vi "ABB Load-Save config.vi"(10 "confirm save":bool, 11 "Mode":enum16{"LOAD", "SAVE"}(ring)) -> ()   [LabVIEW 2017]
uses:
  ABB global.vi
panel:
  out "first row":string[](array[string])
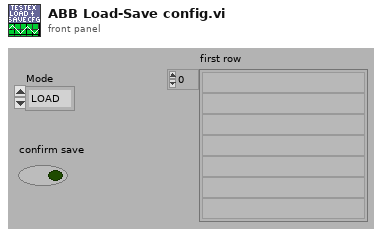
[diagram p1: front panel]
types:
  T1 = cluster{"First row[0]":string, "First row[1]":string, "First row[2]":string, "First row[3]":string}
  T2 = cluster{"First row[0]":string, "First row[1]":string, "First row[2]":string, "First row[3]":string, "First row[4]":string, "First row[5]":string, "First row[6]":string, "First row[7]":string, "First row[8]":string}
  T3 = cluster{"Number Values":i32, "Tolerance":dbl, "Value (ratio) ":dbl[], "Hold time (sec)":dbl}
  T4 = cluster{"Thermal Stability (deg/hr)":dbl, "Reading interval (mins)":dbl}
  T5 = cluster{"Number Values":i32, "Tolerance ":dbl, "Value (ratio)":dbl[], "Hold time (sec)":dbl}
  T6 = cluster{"Simulate Norma":bool, "Norma 5000 Address":u8, "WebDaq IP Address":string, "Simulate cDAQ":bool}
  T7 = cluster{"temp. alloc":i32[], "category":i32[], "Category names":string[], "Category none names":string[]}
  T8 = cluster{"Number of Loads":i32, "Loads (%Rated)":dbl[]}
  T9 = cluster{"VT Primary":dbl, "VT Secondary":dbl, "CT  Primary":dbl, "CT Secondary":dbl, "Current Shunt":enum16{"Internal", "External"}, "Averaging interval":dbl}
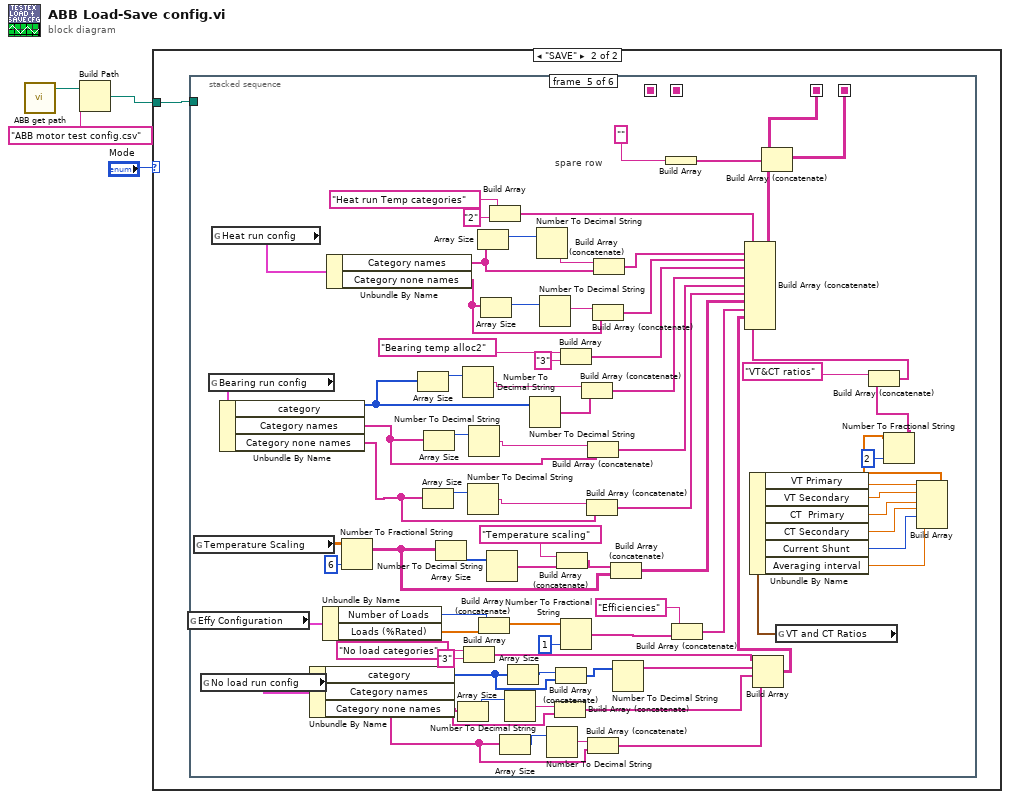
[diagram p0: block diagram]
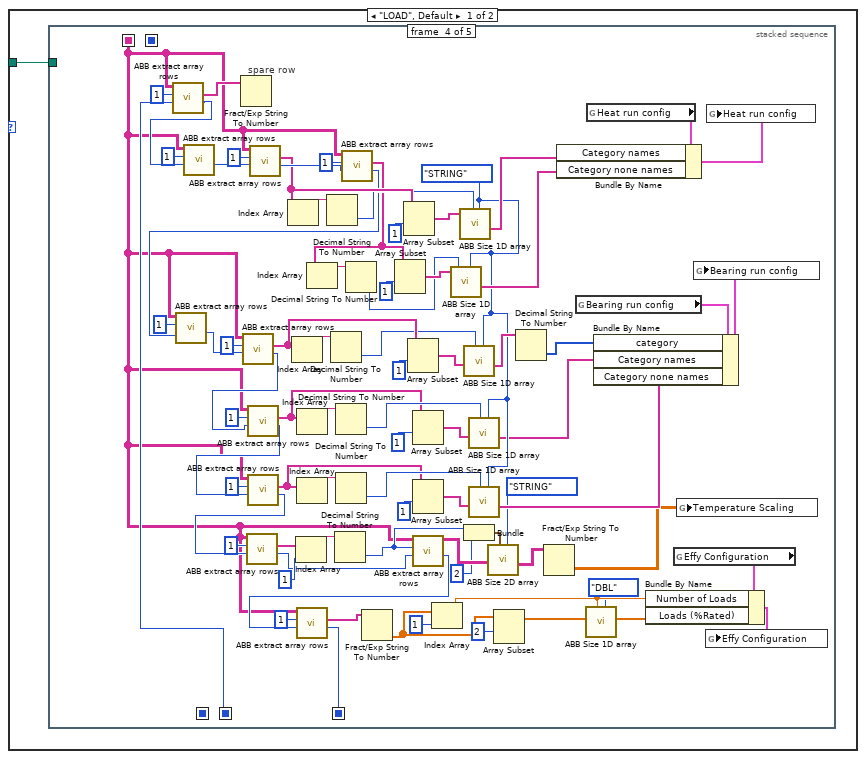
[diagram p2: hidden frame]
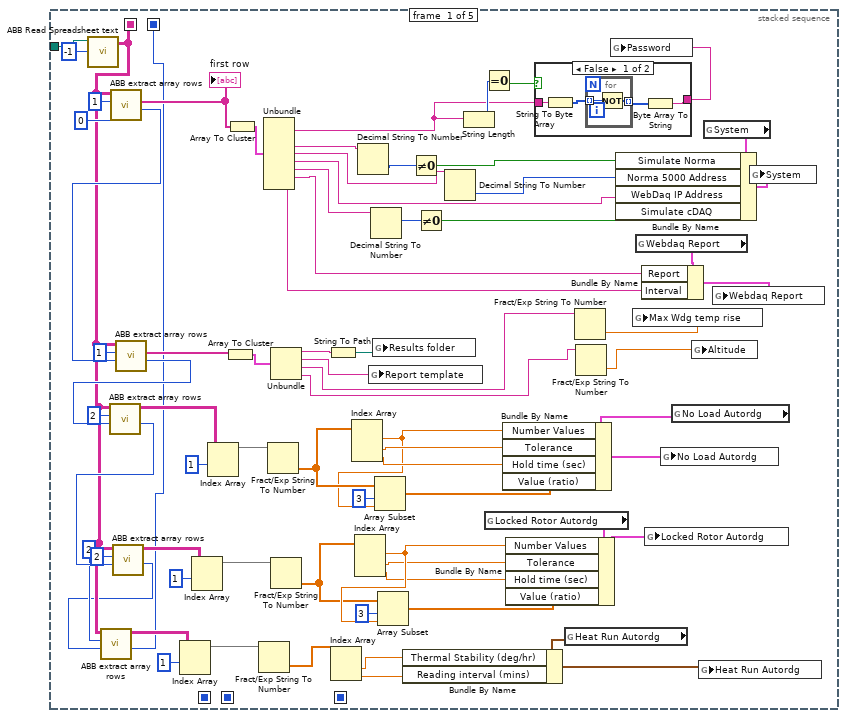
[diagram p3: hidden frame]
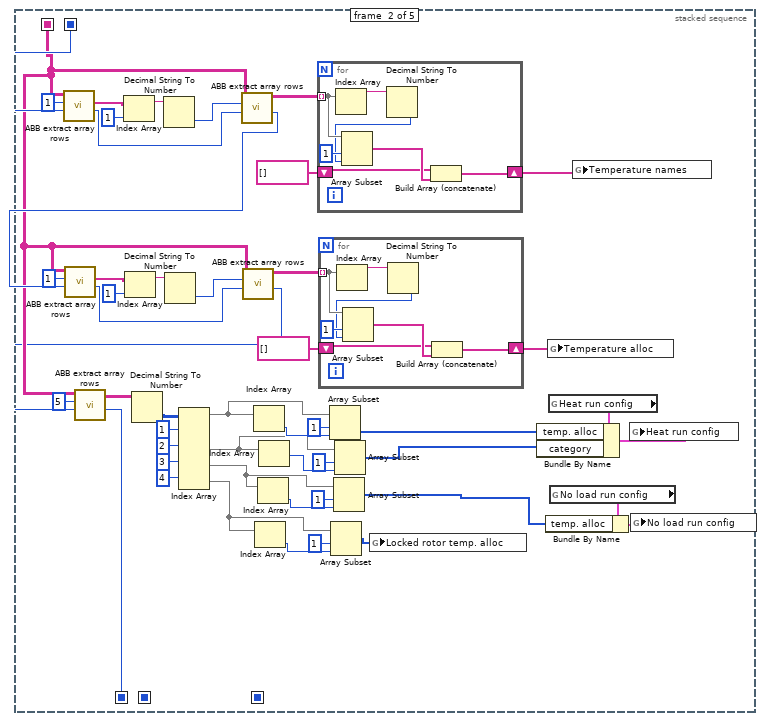
[diagram p5: hidden frame]
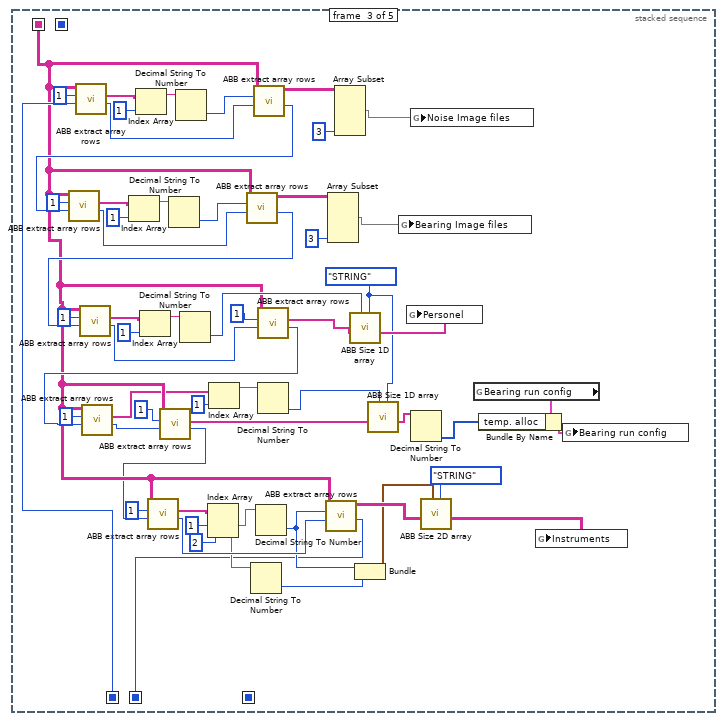
[diagram p6: hidden frame]
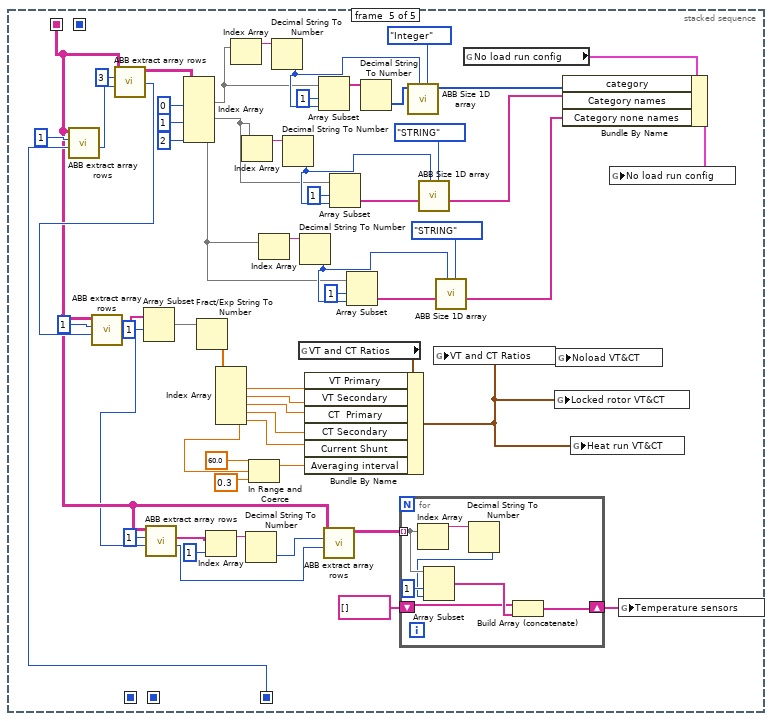
[diagram p7: hidden frame]
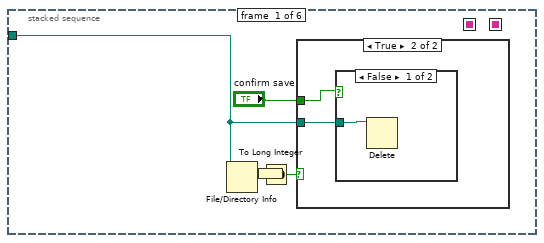
[diagram p8: hidden frame]
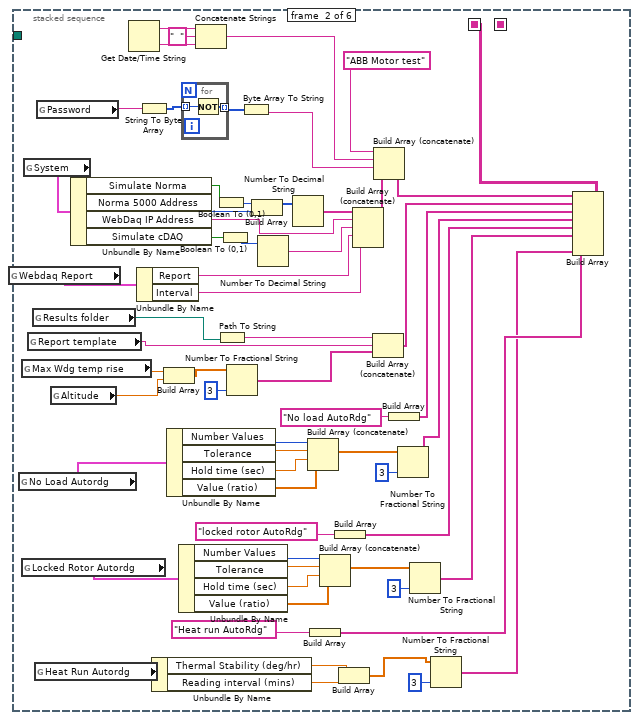
[diagram p11: hidden frame]
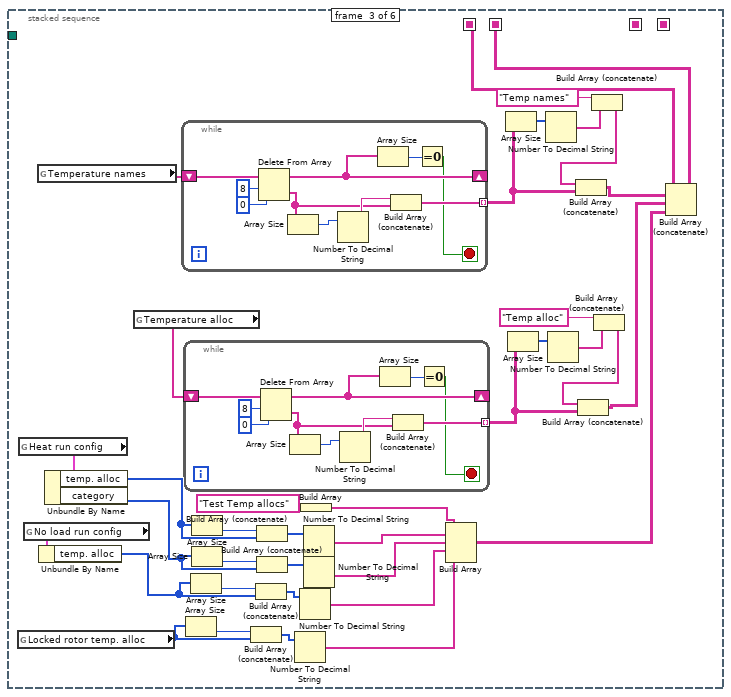
[diagram p12: hidden frame]
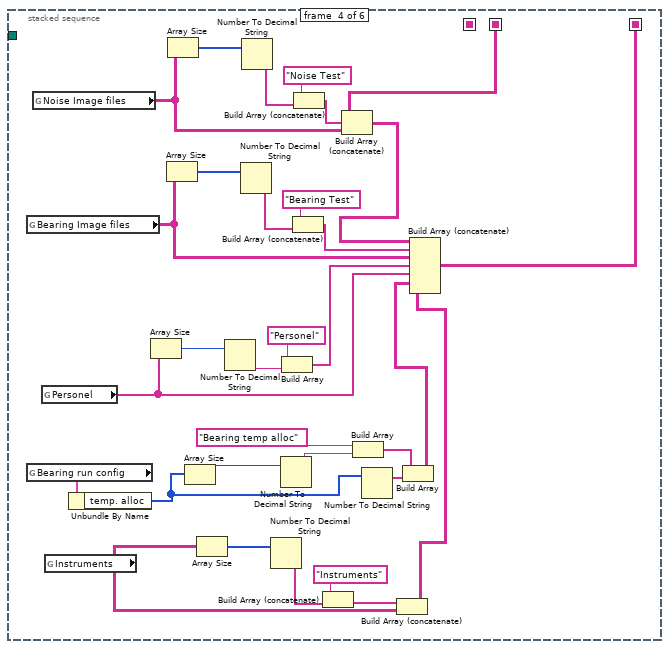
[diagram p13: hidden frame]
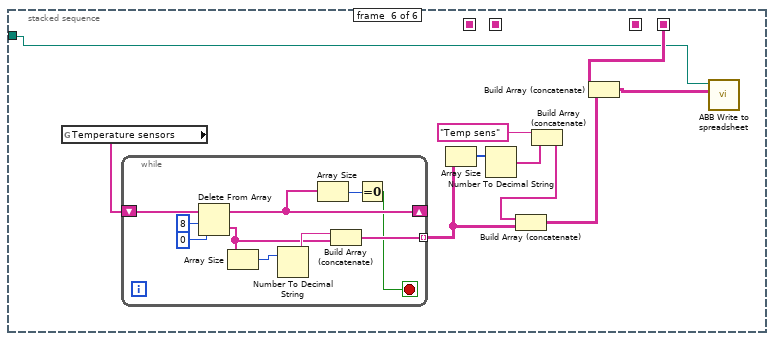
[diagram p14: hidden frame]
diagram:
  n1 = call "ABB get path.vi"() -> ("Path"=w1:path)  [unwired: 11 in]
  n2 = Build Path(base path=w1, name or relative path="ABB motor test config.csv") -> (appended path=w2:path)
  n3 = case shown="\"SAVE\"" "Mode" {
    tunnel: w2 -> [w5 w357]
    frame "LOAD", Default {
      n4 = stacked-sequence {
        seq-local: [w27 _ _ _ _] -> [_ w115 w159 w212 w292]
        seq-local: [w20 _ _ _ _] -> [_ w135 _ _ _]
        seq-local: [_ w100 _ _ _] -> [_ _ w204 _ _]
        seq-local: [_ _ w163 _ _] -> [_ _ _ w289 _]
        seq-local: [_ _ _ w211 _] -> [_ _ _ _ w348]
        tunnel: w5 -> [w74 _ _ _ _]
        frame #0 {
          n5 = call "ABB Read Spreadsheet text.vi"("number of rows (all:-1)"=-1, "file path (dialog if empty)"=w74) -> ("all rows"=w27:string[][])  [unwired: 5 in, 4 out]
          n6 = call "ABB extract array rows.vi"("Row offset"=0, "# rows"=1, "Input array"=w27) -> ("Next row"=w62:i32, "First row"=w71:string[])  [unwired: 6 in, 1 out]
          "first row" <- w71
          n7 = call "ABB extract array rows.vi"("Row offset"=w62, "# rows"=1, "Input array"=w27) -> ("Next row"=w56:i32, "First row"=w61:string[])  [unwired: 6 in, 1 out]
          n8 = call "ABB extract array rows.vi"("Row offset"=w56, "# rows"=2, "Input array"=w27) -> ("Next row"=w32:i32, "All rows"=w55:string[][])  [unwired: 6 in, 1 out]
          n9 = call "ABB extract array rows.vi"("Row offset"=w32, "# rows"=2, "Input array"=w27) -> ("Next row"=w26:i32, "All rows"=w34:string[][])  [unwired: 6 in, 1 out]
          n10 = call "ABB extract array rows.vi"("Row offset"=w26, "# rows"=2, "Input array"=w27) -> ("Next row"=w20:i32, "All rows"=w30:string[][])  [unwired: 6 in, 1 out]
          n11 = Index Array(array=w30, index (row)=1) -> (element=w28:string[])  [unwired: 1 in]
          n12 = Index Array(array=w34, index (row)=1) -> (element=w36:string[])  [unwired: 1 in]
          n13 = Index Array(array=w55, index (row)=1) -> (element=w53:string[])  [unwired: 1 in]
          n14 = Array To Cluster(array=w61) -> (cluster=w60:T1)
          n15 = Array To Cluster(array=w71) -> (cluster=w79:T2)
          n16 = Fract/Exp String To Number(string=w28) -> (number=w24:dbl[])  [unwired: 3 in, 1 out]
          n17 = Unbundle(w79) -> ("First row[2]"=w73:string, "First row[3]"=w69:string, "First row[4]"=w18:string, "First row[5]"=w17:string, "First row[6]"=w16:string, "First row[7]"=w6:string, "First row[8]"=w7:string)  [unwired: 2 out]
          n18 = Fract/Exp String To Number(string=w53) -> (number=w49:dbl[])  [unwired: 3 in, 1 out]
          n19 = Unbundle(w60) -> ("First row[0]"=w59:string, "First row[1]"=w19:string, "First row[2]"=w13:string, "First row[3]"=w12:string)
          n20 = Fract/Exp String To Number(string=w36) -> (number=w40:dbl[])  [unwired: 3 in, 1 out]
          n21 = String To Path(string=w59) -> (path=w58:path)
          n22 = Index Array(array=w24) -> (element #1=w23:dbl, element #2=w22:dbl)  [unwired: 2 in]
          n23 = Index Array(array=w49) -> (element #1=w47:dbl, element #2=w51:dbl, element #3=w50:dbl)  [unwired: 3 in]
          n24 = Index Array(array=w40) -> (element #1=w42:dbl, element #2=w38:dbl, element #3=w39:dbl)  [unwired: 3 in]
          n25 = Decimal String To Number(string=w69) -> (number=w68:i32)  [unwired: 2 in, 1 out]
          n26 = global write "ABB global.vi" "Report template"(w19) -> ()
          n27 = Decimal String To Number(string=w16) -> (number=w15:i32)  [unwired: 2 in, 1 out]
          n28 = global write "ABB global.vi" "Results folder"(w58) -> ()
          n29 = Array Subset(array=w49, index=3, length=w47) -> (w46:dbl[])
          n30 = Array Subset(array=w40, index=3, length=w42) -> (w43:dbl[])
          n31 = Not Equal To 0?(x=w68) -> (x != 0?=w66:bool)
          n32 = Not Equal To 0?(x=w15) -> (x != 0?=w14:bool)
          n33 = Decimal String To Number(string=w18) -> (number=w65:i32)  [unwired: 2 in, 1 out]
          n34 = String Length(string=w73) -> (length=w78:i32)
          n35 = Equal To 0?(x=w78) -> (x = 0?=w77:bool)
          n36 = global read "ABB global.vi" "Locked Rotor Autordg"() -> (w37:T3)
          n37 = Bundle By Name(cluster=w37, "Number Values"=w42, "Tolerance"=w38, "Hold time (sec)"=w39, "Value (ratio)"=w43) -> (w44:T3)
          n38 = case shown="False" w77 {
            tunnel: w73 -> [w81 w86]
            tunnel: [w80 w86] -> w76
            frame False {
              n39 = String To Byte Array(string=w81) -> (unsigned byte array=w83:u8[])
              n40 = for {
                tunnel: w83 -> [w85] mode=indexing
                tunnel: [w84] -> w82 mode=indexing
                n41 = Not(x=w85) -> (.not. x?=w84:u8)
              }
              n42 = Byte Array To String(unsigned byte array=w82) -> (string=w80:string)
            }
            frame True {
            }
          }
          n43 = global read "ABB global.vi" "Heat Run Autordg"() -> (w25:T4)
          n44 = Bundle By Name(cluster=w25, "Thermal Stability (deg/hr)"=w23, "Reading interval (mins)"=w22) -> (w21:T4)
          n45 = Fract/Exp String To Number(string=w13) -> (number=w11:dbl)  [unwired: 3 in, 1 out]
          n46 = Fract/Exp String To Number(string=w12) -> (number=w10:dbl)  [unwired: 3 in, 1 out]
          n47 = global write "ABB global.vi" "Password"(w76) -> ()
          n48 = global write "ABB global.vi" "Max Wdg temp rise"(w11) -> ()
          n49 = global read "ABB global.vi" "Webdaq Report"() -> (w9:cluster{"Report":string, "Interval":string})
          n50 = Bundle By Name(cluster=w9, "Report"=w6, "Interval"=w7) -> (w8:cluster{"Report":string, "Interval":string})
          n51 = global write "ABB global.vi" "Locked Rotor Autordg"(w44) -> ()
          n52 = global read "ABB global.vi" "No Load Autordg"() -> (w52:T5)
          n53 = Bundle By Name(cluster=w52, "Number Values"=w47, "Tolerance"=w51, "Hold time (sec)"=w50, "Value (ratio)"=w46) -> (w45:T5)
          n54 = global write "ABB global.vi" "No Load Autordg"(w45) -> ()
          n55 = global write "ABB global.vi" "Altitude"(w10) -> ()
          n56 = global write "ABB global.vi" "Heat Run Autordg"(w21) -> ()
          n57 = global read "ABB global.vi" "System"() -> (w67:T6)
          n58 = Bundle By Name(cluster=w67, "Simulate Norma"=w66, "Norma 5000 Address"=w65, "WebDaq IP Address"=w17, "Simulate cDAQ"=w14) -> (w64:T6)
          n59 = global write "ABB global.vi" "Webdaq Report"(w8) -> ()
          n60 = global write "ABB global.vi" "System"(w64) -> ()
        }
        frame #1 {
          n61 = call "ABB extract array rows.vi"("Row offset"=w135, "# rows"=1, "Input array"=w115) -> ("Next row"=w131:i32, "First row"=w134:string[])  [unwired: 6 in, 1 out]
          n62 = Index Array(array=w134, index=1) -> (element=w132:string)
          n63 = Decimal String To Number(string=w132) -> (number=w130:i32)  [unwired: 2 in, 1 out]
          n64 = call "ABB extract array rows.vi"("Row offset"=w131, "# rows"=w130, "Input array"=w115) -> ("Next row"=w118:i32, "All rows"=w129:string[][])  [unwired: 6 in, 1 out]
          n65 = call "ABB extract array rows.vi"("Row offset"=w118, "# rows"=1, "Input array"=w115) -> ("Next row"=w123:i32, "First row"=w120:string[])  [unwired: 6 in, 1 out]
          n66 = Index Array(array=w120, index=1) -> (element=w122:string)
          n67 = Decimal String To Number(string=w122) -> (number=w124:i32)  [unwired: 2 in, 1 out]
          n68 = call "ABB extract array rows.vi"("Row offset"=w123, "# rows"=w124, "Input array"=w115) -> ("Next row"=w109:i32, "All rows"=w125:string[][])  [unwired: 6 in, 1 out]
          n69 = call "ABB extract array rows.vi"("Row offset"=w109, "# rows"=5, "Input array"=w115) -> ("Next row"=w100:i32, "All rows"=w114:string[][])  [unwired: 6 in, 1 out]
          n70 = Decimal String To Number(string=w114) -> (number=w113:i32[][])  [unwired: 2 in, 1 out]
          n71 = Index Array(array=w113, index (row) #1=1 ("index (row)"), index (row) #2=2 ("index (row)"), index (row) #3=3 ("index (row)"), index (row) #4=4 ("index (row)")) -> (element #1=w107:i32[], element #2=w94:i32[], element #3=w92:i32[], element #4=w91:i32[])  [unwired: 4 in]
          n72 = Index Array(array=w107) -> (element=w108:i32)  [unwired: 1 in]
          n73 = Index Array(array=w91) -> (element=w103:i32)  [unwired: 1 in]
          n74 = Index Array(array=w92) -> (element=w104:i32)  [unwired: 1 in]
          n75 = Index Array(array=w94) -> (element=w90:i32)  [unwired: 1 in]
          n76 = for {
            tunnel: w129 -> [w150] mode=indexing
            shift-right: [w144] -> w127
            shift-left: string[] [] -> [w145]
            n77 = Index Array(array=w150) -> (element=w148:string)  [unwired: 1 in]
            n78 = Decimal String To Number(string=w148) -> (number=w147:i32)  [unwired: 2 in, 1 out]
            n79 = Array Subset(array=w150, index=1, length=w147) -> (w146:string[])
            n80 = Build Array (concatenate)(w145, w146) -> (w144:string[])
          }
          n81 = for {
            tunnel: w125 -> [w143] mode=indexing
            shift-right: [w137] -> w117
            shift-left: string[] [] -> [w138]
            n82 = Index Array(array=w143) -> (element=w141:string)  [unwired: 1 in]
            n83 = Decimal String To Number(string=w141) -> (number=w140:i32)  [unwired: 2 in, 1 out]
            n84 = Array Subset(array=w143, index=1, length=w140) -> (w139:string[])
            n85 = Build Array (concatenate)(w138, w139) -> (w137:string[])
          }
          n86 = Array Subset(array=w107, index=1, length=w108) -> (w97:i32[])
          n87 = Array Subset(array=w91, index=1, length=w103) -> (w101:i32[])
          n88 = Array Subset(array=w92, index=1, length=w104) -> (w87:i32[])
          n89 = Array Subset(array=w94, index=1, length=w90) -> (w93:i32[])
          n90 = global write "ABB global.vi" "Locked rotor temp. alloc"(w101) -> ()
          n91 = global write "ABB global.vi" "Temperature alloc"(w117) -> ()
          n92 = global read "ABB global.vi" "Heat run config"() -> (w99:T7)
          n93 = Bundle By Name(cluster=w99, "temp. alloc"=w97, "category"=w93) -> (w98:T7)
          n94 = global read "ABB global.vi" "No load run config"() -> (w88:T7)
          n95 = Bundle By Name(cluster=w88, "temp. alloc"=w87) -> (w89:T7)
          n96 = global write "ABB global.vi" "Temperature names"(w127) -> ()
          n97 = global write "ABB global.vi" "Heat run config"(w98) -> ()
          n98 = global write "ABB global.vi" "No load run config"(w89) -> ()
        }
        frame #2 {
          w178 = enum16{"Integer", "DBL", "STRING", "BOOLEAN"}."STRING" ("Type")
          n99 = call "ABB extract array rows.vi"("Row offset"=w204, "# rows"=1, "Input array"=w159) -> ("Next row"=w209:i32, "First row"=w206:string[])  [unwired: 6 in, 1 out]
          n100 = Index Array(array=w206, index=1) -> (element=w208:string)
          n101 = Decimal String To Number(string=w208) -> (number=w210:i32)  [unwired: 2 in, 1 out]
          n102 = call "ABB extract array rows.vi"("Row offset"=w209, "# rows"=w210, "Input array"=w159) -> ("Next row"=w191:i32, "All rows"=w203:string[][])  [unwired: 6 in, 1 out]
          n103 = call "ABB extract array rows.vi"("Row offset"=w191, "# rows"=1, "Input array"=w159) -> ("Next row"=w193:i32, "First row"=w196:string[])  [unwired: 6 in, 1 out]
          n104 = Index Array(array=w196, index=1) -> (element=w194:string)
          n105 = Decimal String To Number(string=w194) -> (number=w192:i32)  [unwired: 2 in, 1 out]
          n106 = call "ABB extract array rows.vi"("Row offset"=w193, "# rows"=w192, "Input array"=w159) -> ("Next row"=w186:i32, "All rows"=w198:string[][])  [unwired: 6 in, 1 out]
          n107 = call "ABB extract array rows.vi"("Row offset"=w186, "# rows"=1, "Input array"=w159) -> ("Next row"=w182:i32, "First row"=w188:string[])  [unwired: 6 in, 1 out]
          n108 = Index Array(array=w188, index=1) -> (element=w190:string)
          n109 = Decimal String To Number(string=w190) -> (number=w179:i32)  [unwired: 2 in, 1 out]
          n110 = call "ABB extract array rows.vi"("Row offset"=w182, "# rows"=1, "Input array"=w159) -> ("Next row"=w184:i32, "First row"=w181:string[])  [unwired: 6 in, 1 out]
          n111 = call "ABB extract array rows.vi"("Row offset"=w184, "# rows"=1, "Input array"=w159) -> ("Next row"=w158:i32, "First row"=w154:string[])  [unwired: 6 in, 1 out]
          n112 = call "ABB extract array rows.vi"("Row offset"=w158, "# rows"=1, "Input array"=w159) -> ("Next row"=w157:i32, "First row"=w155:string[])  [unwired: 6 in, 1 out]
          n113 = call "ABB extract array rows.vi"("Row offset"=w157, "# rows"=1, "Input array"=w159) -> ("Next row"=w176:i32, "First row"=w173:string[])  [unwired: 6 in, 1 out]
          n114 = Index Array(array=w173, index #1=1 ("index"), index #2=2 ("index")) -> (element #1=w175:string, element #2=w168:string)
          n115 = Index Array(array=w154, index=1) -> (element=w152:string)
          n116 = Decimal String To Number(string=w168) -> (number=w166:i32)  [unwired: 2 in, 1 out]
          n117 = Decimal String To Number(string=w175) -> (number=w167:i32)  [unwired: 2 in, 1 out]
          n118 = Decimal String To Number(string=w152) -> (number=w151:i32)  [unwired: 2 in, 1 out]
          n119 = call "ABB extract array rows.vi"("Row offset"=w176, "# rows"=w167, "Input array"=w159) -> ("Next row"=w163:i32, "All rows"=w171:string[][])  [unwired: 6 in, 1 out]
          n120 = Array Subset(array=w198, length (col)=3 ("length")) -> (w200:string[][])  [unwired: 3 in]
          n121 = Array Subset(array=w203, length (col)=3 ("length")) -> (w201:string[][])  [unwired: 3 in]
          n122 = call "ABB Size 1D array.vi"("Type"=w178, "Size"=w179, "String Array in"=w181) -> ("String Array out"=w180:string[])  [unwired: 5 in, 3 out]
          n123 = Bundle(w167, w166) -> (w165:cluster{i32, i32})  [unwired: 1 in]
          n124 = call "ABB Size 1D array.vi"("Type"=w178, "Size"=w151, "String Array in"=w155) -> ("String Array out"=w177:string[])  [unwired: 5 in, 3 out]
          n125 = global write "ABB global.vi" "Bearing Image files"(w200) -> ()
          n126 = global write "ABB global.vi" "Personel"(w180) -> ()
          n127 = global write "ABB global.vi" "Noise Image files"(w201) -> ()
          n128 = Decimal String To Number(string=w177) -> (number=w161:i32[])  [unwired: 2 in, 1 out]
          n129 = call "ABB Size 2D array.vi"("Type"=enum16{"Integer", "DBL", "STRING", "BOOLEAN"}."STRING", "Size"=w165, "String Array in"=w171) -> ("String Array out"=w164:string[][])  [unwired: 5 in, 3 out]
          n130 = global read "ABB global.vi" "Bearing run config"() -> (w162:T7)
          n131 = Bundle By Name(cluster=w162, "temp. alloc"=w161) -> (w160:T7)
          n132 = global write "ABB global.vi" "Instruments"(w164) -> ()
          n133 = global write "ABB global.vi" "Bearing run config"(w160) -> ()
        }
        frame #3 {
          w240 = enum16{"Integer", "DBL", "STRING", "BOOLEAN"}."STRING" ("Type")
          # "spare row"
          n134 = call "ABB extract array rows.vi"("Row offset"=w289, "# rows"=1, "Input array"=w212) -> ("Next row"=w282:i32, "First row"=w288:string[])  [unwired: 6 in, 1 out]
          n135 = call "ABB extract array rows.vi"("Row offset"=w282, "# rows"=1, "Input array"=w212) -> ("Next row"=w281:i32)  [unwired: 6 in, 2 out]
          n136 = Fract/Exp String To Number(string=w288) -> ()  [unwired: 3 in, 2 out]
          n137 = call "ABB extract array rows.vi"("Row offset"=w281, "# rows"=1, "Input array"=w212) -> ("Next row"=w280:i32, "First row"=w278:string[])  [unwired: 6 in, 1 out]
          n138 = Index Array(array=w278) -> (element=w279:string)  [unwired: 1 in]
          n139 = Decimal String To Number(string=w279) -> (number=w274:i32)  [unwired: 2 in, 1 out]
          n140 = call "ABB extract array rows.vi"("Row offset"=w280, "# rows"=1, "Input array"=w212) -> ("Next row"=w262:i32, "First row"=w270:string[])  [unwired: 6 in, 1 out]
          n141 = call "ABB extract array rows.vi"("Row offset"=w262, "# rows"=1, "Input array"=w212) -> ("Next row"=w265:i32)  [unwired: 6 in, 2 out]
          n142 = call "ABB extract array rows.vi"("Row offset"=w265, "# rows"=1, "Input array"=w212) -> ("Next row"=w244:i32, "First row"=w259:string[])  [unwired: 6 in, 1 out]
          n143 = call "ABB extract array rows.vi"("Row offset"=w244, "# rows"=1, "Input array"=w212) -> ("Next row"=w243:i32, "First row"=w242:string[])  [unwired: 6 in, 1 out]
          n144 = call "ABB extract array rows.vi"("Row offset"=w243, "# rows"=1, "Input array"=w212) -> ("Next row"=w234:i32, "First row"=w241:string[])  [unwired: 6 in, 1 out]
          n145 = call "ABB extract array rows.vi"("Row offset"=w234, "# rows"=1, "Input array"=w212) -> ("Next row"=w232:i32, "First row"=w237:string[])  [unwired: 6 in, 1 out]
          n146 = Index Array(array=w259) -> (element=w257:string)  [unwired: 1 in]
          n147 = Index Array(array=w237, index=1) -> (element=w236:string)
          n148 = Index Array(array=w242) -> (element=w254:string)  [unwired: 1 in]
          n149 = Index Array(array=w241) -> (element=w245:string)  [unwired: 1 in]
          n150 = Index Array(array=w270) -> (element=w271:string)  [unwired: 1 in]
          n151 = Decimal String To Number(string=w257) -> (number=w258:i32)  [unwired: 2 in, 1 out]
          n152 = Decimal String To Number(string=w236) -> (number=w229:i32)  [unwired: 2 in, 1 out]
          n153 = Decimal String To Number(string=w254) -> (number=w253:i32)  [unwired: 2 in, 1 out]
          n154 = Decimal String To Number(string=w245) -> (number=w246:i32)  [unwired: 2 in, 1 out]
          n155 = Decimal String To Number(string=w271) -> (number=w269:i32)  [unwired: 2 in, 1 out]
          n156 = Array Subset(array=w270, index=1) -> (w273:string[])  [unwired: 1 in]
          n157 = Array Subset(array=w278, index=1) -> (w276:string[])  [unwired: 1 in]
          n158 = Array Subset(array=w259, index=1) -> (w261:string[])  [unwired: 1 in]
          n159 = Array Subset(array=w242, index=1) -> (w251:string[])  [unwired: 1 in]
          n160 = Array Subset(array=w241, index=1) -> (w248:string[])  [unwired: 1 in]
          n161 = call "ABB extract array rows.vi"("Row offset"=w232, "# rows"=w229, "Input array"=w212) -> ("Next row"=w223:i32, "All rows"=w231:string[][])  [unwired: 6 in, 1 out]
          n162 = call "ABB extract array rows.vi"("Row offset"=w223, "# rows"=1, "Input array"=w212) -> ("Next row"=w211:i32, "First row"=w222:string[])  [unwired: 6 in, 1 out]
          n163 = Fract/Exp String To Number(string=w222) -> (number=w220:dbl[])  [unwired: 3 in, 1 out]
          n164 = Index Array(array=w220, index=1) -> (element=w216:dbl)
          n165 = call "ABB Size 1D array.vi"("Type"=w240, "Size"=w269, "String Array in"=w273) -> ("String Array out"=w268:string[])  [unwired: 5 in, 3 out]
          n166 = call "ABB Size 1D array.vi"("Type"=w240, "Size"=w274, "String Array in"=w276) -> ("String Array out"=w275:string[])  [unwired: 5 in, 3 out]
          n167 = call "ABB Size 1D array.vi"("Type"=w240, "Size"=w258, "String Array in"=w261) -> ("String Array out"=w256:string[])  [unwired: 5 in, 3 out]
          n168 = Bundle(w229, 2) -> (w227:cluster{i32, i32})  [unwired: 1 in]
          n169 = call "ABB Size 1D array.vi"("Type"=w240, "Size"=w253, "String Array in"=w251) -> ("String Array out"=w238:string[])  [unwired: 5 in, 3 out]
          n170 = call "ABB Size 1D array.vi"("Type"=w240, "Size"=w246, "String Array in"=w248) -> ("String Array out"=w239:string[])  [unwired: 5 in, 3 out]
          n171 = call "ABB Size 2D array.vi"("Type"=enum16{"Integer", "DBL", "STRING", "BOOLEAN"}."STRING", "Size"=w227, "String Array in"=w231) -> ("String Array out"=w226:string[][])  [unwired: 5 in, 3 out]
          n172 = Array Subset(array=w220, index=2) -> (w217:dbl[])  [unwired: 1 in]
          n173 = Decimal String To Number(string=w256) -> (number=w255:i32[])  [unwired: 2 in, 1 out]
          n174 = Fract/Exp String To Number(string=w226) -> (number=w225:dbl[][])  [unwired: 3 in, 1 out]
          n175 = global read "ABB global.vi" "Bearing run config"() -> (w267:T7)
          n176 = call "ABB Size 1D array.vi"("Type"=enum16{"Integer", "DBL", "STRING", "BOOLEAN"}."DBL", "Size"=w216, "DBL Array In"=w217) -> ("DBL Array out"=w213:dbl[])  [unwired: 5 in, 3 out]
          n177 = global read "ABB global.vi" "Heat run config"() -> (w287:T7)
          n178 = Bundle By Name(cluster=w287, "Category names"=w275, "Category none names"=w268) -> (w286:T7)
          n179 = Bundle By Name(cluster=w267, "category"=w255, "Category names"=w238, "Category none names"=w239) -> (w266:T7)
          n180 = global read "ABB global.vi" "Effy Configuration"() -> (w218:T8)
          n181 = Bundle By Name(cluster=w218, "Number of Loads"=w216, "Loads (%Rated)"=w213) -> (w214:T8)
          n182 = global write "ABB global.vi" "Temperature Scaling"(w225) -> ()
          n183 = global write "ABB global.vi" "Bearing run config"(w266) -> ()
          n184 = global write "ABB global.vi" "Effy Configuration"(w214) -> ()
          n185 = global write "ABB global.vi" "Heat run config"(w286) -> ()
        }
        frame #4 {
          n186 = call "ABB extract array rows.vi"("Row offset"=w348, "# rows"=1, "Input array"=w292) -> ("Next row"=w346:i32)  [unwired: 6 in, 2 out]
          n187 = call "ABB extract array rows.vi"("Row offset"=w346, "# rows"=3, "Input array"=w292) -> ("Next row"=w316:i32, "All rows"=w336:string[][])  [unwired: 6 in, 1 out]
          n188 = call "ABB extract array rows.vi"("Row offset"=w316, "# rows"=1, "Input array"=w292) -> ("Next row"=w291:i32, "First row"=w308:string[])  [unwired: 6 in, 1 out]
          n189 = Array Subset(array=w308, index=1) -> (w309:string[])  [unwired: 1 in]
          n190 = call "ABB extract array rows.vi"("Row offset"=w291, "# rows"=1, "Input array"=w292) -> ("Next row"=w298:i32, "First row"=w295:string[])  [unwired: 6 in, 1 out]
          n191 = Index Array(array=w336, index (row) #1=0 ("index (row)"), index (row) #2=1 ("index (row)"), index (row) #3=2 ("index (row)")) -> (element #1=w335:string[], element #2=w323:string[], element #3=w318:string[])  [unwired: 3 in]
          n192 = Fract/Exp String To Number(string=w309) -> (number=w314:dbl[])  [unwired: 3 in, 1 out]
          n193 = Index Array(array=w295, index=1) -> (element=w297:string)
          n194 = Index Array(array=w314) -> (element #1=w313:dbl, element #2=w312:dbl, element #3=w311:dbl, element #4=w310:dbl, element #5=w305:dbl)  [unwired: 5 in]
          n195 = Index Array(array=w335) -> (element=w345:string)  [unwired: 1 in]
          n196 = Index Array(array=w323) -> (element=w328:string)  [unwired: 1 in]
          n197 = Decimal String To Number(string=w297) -> (number=w299:i32)  [unwired: 2 in, 1 out]
          n198 = In Range and Coerce(upper limit=60.0, x=w305, lower limit=0.3) -> (coerced(x)=w304:dbl)  [unwired: 1 out]
          n199 = Index Array(array=w318) -> (element=w327:string)  [unwired: 1 in]
          n200 = Decimal String To Number(string=w345) -> (number=w337:i32)  [unwired: 2 in, 1 out]
          n201 = Decimal String To Number(string=w328) -> (number=w331:i32)  [unwired: 2 in, 1 out]
          n202 = global read "ABB global.vi" "VT and CT Ratios"() -> (w315:T9)
          n203 = Decimal String To Number(string=w327) -> (number=w324:i32)  [unwired: 2 in, 1 out]
          n204 = Bundle By Name(cluster=w315, "VT Primary"=w313, "VT Secondary"=w312, "CT  Primary"=w311, "CT Secondary"=w310, "Current Shunt"=w305, "Averaging interval"=w304) -> (w302:T9)
          n205 = Array Subset(array=w335, index=1, length=w337) -> (w341:string[])
          n206 = call "ABB extract array rows.vi"("Row offset"=w298, "# rows"=w299, "Input array"=w292) -> ("All rows"=w300:string[][])  [unwired: 6 in, 2 out]
          n207 = Array Subset(array=w323, index=1, length=w331) -> (w322:string[])
          n208 = Array Subset(array=w318, index=1, length=w324) -> (w320:string[])
          n209 = Decimal String To Number(string=w341) -> (number=w340:i32[])  [unwired: 2 in, 1 out]
          n210 = for {
            tunnel: w300 -> [w356] mode=indexing
            shift-right: [w350] -> w293
            shift-left: string[] [] -> [w351]
            n211 = Index Array(array=w356) -> (element=w354:string)  [unwired: 1 in]
            n212 = Decimal String To Number(string=w354) -> (number=w353:i32)  [unwired: 2 in, 1 out]
            n213 = Array Subset(array=w356, index=1, length=w353) -> (w352:string[])
            n214 = Build Array (concatenate)(w351, w352) -> (w350:string[])
          }
          n215 = call "ABB Size 1D array.vi"("Type"=enum16{"Integer", "DBL", "STRING", "BOOLEAN"}."Integer", "Size"=w337, "Integer Array In"=w340) -> ("Integer Array Out"=w339:i32[])  [unwired: 5 in, 3 out]
          n216 = call "ABB Size 1D array.vi"("Type"=enum16{"Integer", "DBL", "STRING", "BOOLEAN"}."STRING", "Size"=w331, "String Array in"=w322) -> ("String Array out"=w321:string[])  [unwired: 5 in, 3 out]
          n217 = global write "ABB global.vi" "VT and CT Ratios"(w302) -> ()
          n218 = call "ABB Size 1D array.vi"("Type"=enum16{"Integer", "DBL", "STRING", "BOOLEAN"}."STRING", "Size"=w324, "String Array in"=w320) -> ("String Array out"=w319:string[])  [unwired: 5 in, 3 out]
          n219 = global read "ABB global.vi" "No load run config"() -> (w343:T7)
          n220 = global write "ABB global.vi" "Locked rotor VT&CT"(w302) -> ()
          n221 = global write "ABB global.vi" "Noload VT&CT"(w302) -> ()
          n222 = Bundle By Name(cluster=w343, "category"=w339, "Category names"=w321, "Category none names"=w319) -> (w342:T7)
          n223 = global write "ABB global.vi" "Heat run VT&CT"(w302) -> ()
          n224 = global write "ABB global.vi" "No load run config"(w342) -> ()
          n225 = global write "ABB global.vi" "Temperature sensors"(w293) -> ()
        }
      }
    }
    frame "SAVE" {
      n226 = stacked-sequence {
        seq-local: [_ w417 _ _ _ _] -> [_ _ w460 _ _ _]
        seq-local: [_ _ w458 _ _ _] -> [_ _ _ w513 _ _]
        seq-local: [_ _ _ w489 _ _] -> [_ _ _ _ w597 _]
        seq-local: [_ _ _ _ w519 _] -> [_ _ _ _ _ w607]
        tunnel: w357 -> [w359 _ _ _ _ w599]
        frame #0 {
          n227 = File/Directory Info(path=w359) -> (size=w358:i64)  [unwired: 1 in, 6 out]
          n228 = To Long Integer(number=w358) -> (32bit integer=w362:i32)
          n229 = Not Equal To 0?(x=w362) -> (x != 0?=w361:bool)
          n230 = case shown="True" w361 {
            tunnel: "confirm save" -> [_ w364]
            tunnel: w359 -> [_ w363]
            frame False {
            }
            frame True {
              n231 = case shown="False" w364 {
                tunnel: w363 -> [w365 _]
                frame False {
                  n232 = Delete(path (use dialog)=w365) -> ()  [unwired: 4 in, 3 out]
                }
                frame True {
                }
              }
            }
          }
        }
        frame #1 {
          n233 = global read "ABB global.vi" "Webdaq Report"() -> (w368:cluster{"Report":string, "Interval":string})
          n234 = global read "ABB global.vi" "No Load Autordg"() -> (w407:T5)
          n235 = global read "ABB global.vi" "Max Wdg temp rise"() -> (w373:dbl)
          n236 = global read "ABB global.vi" "Locked Rotor Autordg"() -> (w390:T3)
          n237 = global read "ABB global.vi" "System"() -> (w416:T6)
          n238 = global read "ABB global.vi" "Report template"() -> (w379:string)
          n239 = global read "ABB global.vi" "Results folder"() -> (w410:path)
          n240 = global read "ABB global.vi" "Heat Run Autordg"() -> (w387:T4)
          n241 = global read "ABB global.vi" "Password"() -> (w425:string)
          n242 = global read "ABB global.vi" "Altitude"() -> (w372:dbl)
          n243 = Unbundle By Name(w416) -> ("Simulate Norma"=w415:bool, "Norma 5000 Address"=w413:u8, "WebDaq IP Address"=w377:string, "Simulate cDAQ"=w376:bool)
          n244 = Get Date/Time String() -> (date string=w423:string, time string=w422:string)  [unwired: 3 in]
          n245 = Unbundle By Name(w368) -> ("Report"=w367:string, "Interval"=w366:string)
          n246 = String To Byte Array(string=w425) -> (unsigned byte array=w427:u8[])
          n247 = Unbundle By Name(w387) -> ("Thermal Stability (deg/hr)"=w385:dbl, "Reading interval (mins)"=w384:dbl)
          n248 = Build Array(w373, w372) -> (w371:dbl[])
          n249 = Unbundle By Name(w407) -> ("Number Values"=w406:i32, "Tolerance"=w405:dbl, "Hold time (sec)"=w402:dbl, "Value (ratio)"=w401:dbl[])
          n250 = Unbundle By Name(w390) -> ("Number Values"=w391:i32, "Tolerance"=w392:dbl, "Hold time (sec)"=w395:dbl, "Value (ratio)"=w396:dbl[])
          n251 = for {
            tunnel: w427 -> [w429] mode=indexing
            tunnel: [w428] -> w426 mode=indexing
            n252 = Not(x=w429) -> (.not. x?=w428:u8)
          }
          n253 = Concatenate Strings(w423, "  " ("string"), w422) -> (w420:string)
          n254 = Boolean To (0,1)(Boolean=w415) -> (0, 1=w414:i16)
          n255 = Path To String(path=w410) -> (string=w408:string)
          n256 = Boolean To (0,1)(Boolean=w376) -> (0, 1=w375:i16)
          n257 = Number To Fractional String(number=w371, precision (6)=i16 3) -> (F-format string=w369:string[])  [unwired: 2 in]
          n258 = Byte Array To String(unsigned byte array=w426) -> (string=w424:string)
          n259 = Build Array(w414, w413) -> (w412:i16[])
          n260 = Number To Decimal String(number=w375) -> (decimal integer string=w374:string)  [unwired: 1 in]
          n261 = Number To Decimal String(number=w412) -> (decimal integer string=w411:string[])  [unwired: 1 in]
          n262 = Build Array (concatenate)(w406, w405, w402, w401) -> (w404:dbl[])
          n263 = Build Array("Heat run AutoRdg") -> (w383:string[])
          n264 = Build Array (concatenate)(w391, w392, w395, w396) -> (w393:dbl[])
          n265 = Build Array("locked rotor AutoRdg") -> (w389:string[])
          n266 = Build Array(w385, w384) -> (w381:dbl[])
          n267 = Build Array (concatenate)(w411, w377, w374, w367, w366) -> (w378:string[])
          n268 = Build Array (concatenate)(w408, w379, w369) -> (w409:string[])
          n269 = Build Array (concatenate)("ABB Motor test", w420, w424, w378) -> (w418:string[])
          n270 = Build Array("No load AutoRdg") -> (w399:string[])
          n271 = Number To Fractional String(number=w404, precision (6)=i16 3) -> (F-format string=w398:string[])  [unwired: 2 in]
          n272 = Number To Fractional String(number=w393, precision (6)=i16 3) -> (F-format string=w388:string[])  [unwired: 2 in]
          n273 = Number To Fractional String(number=w381, precision (6)=i16 3) -> (F-format string=w380:string[])  [unwired: 2 in]
          n274 = Build Array(w418, w409, w399, w398, w389, w388, w383, w380) -> (w417:string[][])
        }
        frame #2 {
          n275 = global read "ABB global.vi" "Locked rotor temp. alloc"() -> (w441:i32[])
          n276 = global read "ABB global.vi" "Heat run config"() -> (w437:T7)
          n277 = global read "ABB global.vi" "No load run config"() -> (w431:T7)
          n278 = global read "ABB global.vi" "Temperature names"() -> (w466:string[])
          n279 = Unbundle By Name(w431) -> ("temp. alloc"=w430:i32[])
          n280 = Unbundle By Name(w437) -> ("temp. alloc"=w436:i32[], "category"=w433:i32[])
          n281 = global read "ABB global.vi" "Temperature alloc"() -> (w452:string[])
          n282 = while {
            shift-right: [w480] -> _
            shift-left: w466 -> [w486]
            tunnel: [w481] -> w461 mode=indexing
            stop <- w478 stop-if-true
            n283 = Delete From Array(array=w486, length=8, index=0) -> (deleted portion=w482:string[], array with subset deleted=w480:string[])
            n284 = Array Size(array=w482) -> (size(s)=w484:i32)
            n285 = Number To Decimal String(number=w484) -> (decimal integer string=w483:string)  [unwired: 1 in]
            n286 = Array Size(array=w480) -> (size(s)=w479:i32)
            n287 = Build Array (concatenate)(w483, w482) -> (w481:string[])
            n288 = Equal To 0?(x=w479) -> (x = 0?=w478:bool)
          }
          n289 = while {
            shift-right: [w470] -> _
            shift-left: w452 -> [w476]
            tunnel: [w471] -> w457 mode=indexing
            stop <- w468 stop-if-true
            n290 = Delete From Array(array=w476, length=8, index=0) -> (deleted portion=w472:string[], array with subset deleted=w470:string[])
            n291 = Array Size(array=w472) -> (size(s)=w474:i32)
            n292 = Number To Decimal String(number=w474) -> (decimal integer string=w473:string)  [unwired: 1 in]
            n293 = Array Size(array=w470) -> (size(s)=w469:i32)
            n294 = Build Array (concatenate)(w473, w472) -> (w471:string[])
            n295 = Equal To 0?(x=w469) -> (x = 0?=w468:bool)
          }
          n296 = Array Size(array=w441) -> (size(s)=w442:i32)
          n297 = Array Size(array=w430) -> (size(s)=w445:i32)
          n298 = Array Size(array=w436) -> (size(s)=w446:i32)
          n299 = Array Size(array=w433) -> (size(s)=w435:i32)
          n300 = Build Array (concatenate)(w442, w441) -> (w443:i32[])
          n301 = Build Array (concatenate)(w445, w430) -> (w444:i32[])
          n302 = Build Array (concatenate)(w446, w436) -> (w447:i32[])
          n303 = Build Array (concatenate)(w435, w433) -> (w434:i32[])
          n304 = Number To Decimal String(number=w443) -> (decimal integer string=w439:string[])  [unwired: 1 in]
          n305 = Number To Decimal String(number=w444) -> (decimal integer string=w440:string[])  [unwired: 1 in]
          n306 = Build Array("Test Temp allocs") -> (w449:string[])
          n307 = Number To Decimal String(number=w447) -> (decimal integer string=w448:string[])  [unwired: 1 in]
          n308 = Number To Decimal String(number=w434) -> (decimal integer string=w432:string[])  [unwired: 1 in]
          n309 = Build Array(w449, w448, w432, w440, w439) -> (w438:string[][])
          n310 = Array Size(array=w461) -> (size(s)=w465:i32[])
          n311 = Array Size(array=w457) -> (size(s)=w453:i32[])
          n312 = Number To Decimal String(number=w465) -> (decimal integer string=w463:string[])  [unwired: 1 in]
          n313 = Number To Decimal String(number=w453) -> (decimal integer string=w455:string[])  [unwired: 1 in]
          n314 = Build Array (concatenate)("Temp names", w463) -> (w462:string[])
          n315 = Build Array (concatenate)(w462, w461) -> (w459:string[][])
          n316 = Build Array (concatenate)("Temp alloc", w455) -> (w456:string[])
          n317 = Build Array (concatenate)(w456, w457) -> (w451:string[][])
          n318 = Build Array (concatenate)(w460, w459, w451, w438) -> (w458:string[][])
        }
        frame #3 {
          n319 = global read "ABB global.vi" "Bearing Image files"() -> (w512:string[][])
          n320 = global read "ABB global.vi" "Bearing run config"() -> (w488:T7)
          n321 = global read "ABB global.vi" "Noise Image files"() -> (w514:string[][])
          n322 = global read "ABB global.vi" "Personel"() -> (w502:string[])
          n323 = global read "ABB global.vi" "Instruments"() -> (w491:string[][])
          n324 = Unbundle By Name(w488) -> ("temp. alloc"=w487:i32[])
          n325 = Array Size(array=w502) -> (size(s)=w506:i32)
          n326 = Array Size(array=w512) -> (size(s)=w508:i32[])
          n327 = Array Size(array=w514) -> (size(s)=w518:i32[])
          n328 = Array Size(array=w487) -> (size(s)=w498:i32)
          n329 = Array Size(array=w491) -> (size(s)=w495:i32[])
          n330 = Number To Decimal String(number=w506) -> (decimal integer string=w505:string)  [unwired: 1 in]
          n331 = Number To Decimal String(number=w508) -> (decimal integer string=w509:string[])  [unwired: 1 in]
          n332 = Number To Decimal String(number=w518) -> (decimal integer string=w517:string[])  [unwired: 1 in]
          n333 = Number To Decimal String(number=w495) -> (decimal integer string=w494:string[])  [unwired: 1 in]
          n334 = Number To Decimal String(number=w498) -> (decimal integer string=w500:string)  [unwired: 1 in]
          n335 = Build Array("Personel", w505) -> (w503:string[])
          n336 = Build Array (concatenate)("Bearing Test", w509) -> (w511:string[])
          n337 = Build Array (concatenate)("Noise Test", w517) -> (w515:string[])
          n338 = Build Array (concatenate)("Instruments", w494) -> (w492:string[])
          n339 = Build Array (concatenate)(w513, w515, w514) -> (w507:string[][])
          n340 = Build Array("Bearing temp alloc", w500) -> (w499:string[])
          n341 = Number To Decimal String(number=w487) -> (decimal integer string=w497:string[])  [unwired: 1 in]
          n342 = Build Array (concatenate)(w492, w491) -> (w490:string[][])
          n343 = Build Array(w499, w497) -> (w496:string[][])
          n344 = Build Array (concatenate)(w507, w511, w512, w503, w502, w496, w490) -> (w489:string[][])
        }
        frame #4 {
          # "spare row"
          n345 = global read "ABB global.vi" "Effy Configuration"() -> (w558:T8)
          n346 = global read "ABB global.vi" "Temperature Scaling"() -> (w566:dbl[][])
          n347 = global read "ABB global.vi" "No load run config"() -> (w550:T7)
          n348 = global read "ABB global.vi" "Bearing run config"() -> (w580:T7)
          n349 = global read "ABB global.vi" "Heat run config"() -> (w595:T7)
          n350 = Unbundle By Name(w580) -> ("category"=w581:i32[], "Category names"=w572:string[], "Category none names"=w571:string[])
          n351 = Unbundle By Name(w550) -> ("category"=w546:i32[], "Category names"=w545:string[], "Category none names"=w542:string[])
          n352 = Unbundle By Name(w558) -> ("Number of Loads"=w557:i32, "Loads (%Rated)"=w556:dbl[])
          n353 = Unbundle By Name(w595) -> ("Category names"=w592:string[], "Category none names"=w589:string[])
          n354 = Number To Fractional String(number=w566, precision (6)=i16 6) -> (F-format string=w560:string[][])  [unwired: 2 in]
          n355 = Array Size(array=w581) -> (size(s)=w582:i32)
          n356 = Array Size(array=w571) -> (size(s)=w574:i32)
          n357 = Array Size(array=w572) -> (size(s)=w575:i32)
          n358 = Array Size(array=w560) -> (size(s)=w564:i32[])
          n359 = Array Size(array=w545) -> (size(s)=w538:i32)
          n360 = Number To Decimal String(number=w582) -> (decimal integer string=w578:string)  [unwired: 1 in]
          n361 = Build Array("No load categories", "3" ("element")) -> (w544:string[])
          n362 = Number To Decimal String(number=w574) -> (decimal integer string=w573:string)  [unwired: 1 in]
          n363 = Number To Decimal String(number=w575) -> (decimal integer string=w576:string)  [unwired: 1 in]
          n364 = Array Size(array=w592) -> (size(s)=w594:i32)
          n365 = Build Array (concatenate)(w557, w556) -> (w555:dbl[])
          n366 = Array Size(array=w589) -> (size(s)=w590:i32)
          n367 = Number To Decimal String(number=w564) -> (decimal integer string=w563:string[])  [unwired: 1 in]
          n368 = Build Array("Heat run Temp categories", "2" ("element")) -> (w587:string[])
          n369 = Array Size(array=w542) -> (size(s)=w541:i32)
          n370 = Number To Decimal String(number=w538) -> (decimal integer string=w537:string)  [unwired: 1 in]
          n371 = Array Size(array=w546) -> (size(s)=w547:i32)
          n372 = Number To Decimal String(number=w581) -> (decimal integer string=w577:string[])  [unwired: 1 in]
          n373 = Number To Decimal String(number=w594) -> (decimal integer string=w593:string)  [unwired: 1 in]
          n374 = Number To Decimal String(number=w590) -> (decimal integer string=w591:string)  [unwired: 1 in]
          n375 = Number To Decimal String(number=w541) -> (decimal integer string=w540:string)  [unwired: 1 in]
          n376 = Build Array (concatenate)(w537, w545) -> (w534:string[])
          n377 = Build Array (concatenate)(w547, w546) -> (w536:i32[])
          n378 = Build Array (concatenate)("Temperature scaling", w563) -> (w561:string[])
          n379 = Build Array("Bearing temp alloc2", "3" ("element")) -> (w570:string[])
          n380 = Number To Fractional String(number=w555, precision (6)=i16 1) -> (F-format string=w553:string[])  [unwired: 2 in]
          n381 = Build Array (concatenate)(w578, w577) -> (w569:string[])
          n382 = Build Array (concatenate)(w573, w571) -> (w567:string[])
          n383 = Build Array (concatenate)(w576, w572) -> (w568:string[])
          n384 = Build Array (concatenate)(w540, w542) -> (w535:string[])
          n385 = Build Array (concatenate)(w591, w589) -> (w585:string[])
          n386 = Build Array (concatenate)(w593, w592) -> (w586:string[])
          n387 = Build Array (concatenate)(w561, w560) -> (w559:string[][])
          n388 = Number To Decimal String(number=w536) -> (decimal integer string=w543:string[])  [unwired: 1 in]
          n389 = Build Array("") -> (w532:string[])
          n390 = Build Array (concatenate)("Efficiencies", w553) -> (w552:string[])
          n391 = Build Array(w544, w543, w534, w535) -> (w539:string[][])
          n392 = global read "ABB global.vi" "VT and CT Ratios"() -> (w531:T9)
          n393 = Unbundle By Name(w531) -> ("VT Primary"=w530:dbl, "VT Secondary"=w529:dbl, "CT  Primary"=w528:dbl, "CT Secondary"=w527:dbl, "Current Shunt"=w526:enum16{"Internal", "External"}, "Averaging interval"=w520:dbl)
          n394 = Build Array(w530, w529, w528, w527, w526, w520) -> (w525:dbl[])
          n395 = Number To Fractional String(number=w525, precision (6)=i16 2) -> (F-format string=w522:string[])  [unwired: 2 in]
          n396 = Build Array (concatenate)("VT&CT ratios", w522) -> (w523:string[])
          n397 = Build Array (concatenate)(w587, w586, w585, w570, w569, w568, w567, w559, w552, w539, w523) -> (w584:string[][])
          n398 = Build Array (concatenate)(w597, w532, w584) -> (w519:string[][])
        }
        frame #5 {
          n399 = global read "ABB global.vi" "Temperature sensors"() -> (w601:string[])
          n400 = while {
            shift-right: [w611] -> _
            shift-left: w601 -> [w617]
            tunnel: [w612] -> w606 mode=indexing
            stop <- w609 stop-if-true
            n401 = Delete From Array(array=w617, length=8, index=0) -> (deleted portion=w613:string[], array with subset deleted=w611:string[])
            n402 = Array Size(array=w613) -> (size(s)=w615:i32)
            n403 = Number To Decimal String(number=w615) -> (decimal integer string=w614:string)  [unwired: 1 in]
            n404 = Array Size(array=w611) -> (size(s)=w610:i32)
            n405 = Build Array (concatenate)(w614, w613) -> (w612:string[])
            n406 = Equal To 0?(x=w610) -> (x = 0?=w609:bool)
          }
          n407 = Array Size(array=w606) -> (size(s)=w602:i32[])
          n408 = Number To Decimal String(number=w602) -> (decimal integer string=w604:string[])  [unwired: 1 in]
          n409 = Build Array (concatenate)("Temp sens", w604) -> (w605:string[])
          n410 = Build Array (concatenate)(w605, w606) -> (w600:string[][])
          n411 = Build Array (concatenate)(w607, w600) -> (w598:string[][])
          n412 = call "ABB Write to spreadsheet.vi"("2D data"=w598, "file path (dialog if empty)"=w599) -> ()  [unwired: 6 in, 1 out]
        }
      }
    }
  }
